vi "Example1 Chap1.vi"() -> ()   [LabVIEW 2013]
panel:
  in  "stop":bool
  out "Gauge":i32(knob) scale=0.0..10.0
  in  "Start":bool
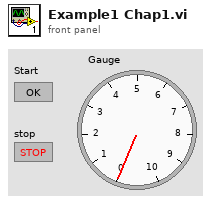
[diagram p1: front panel]
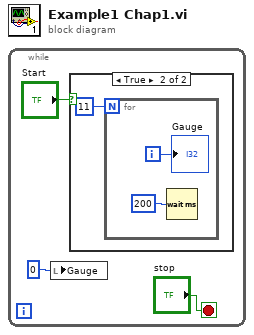
[diagram p0: block diagram]
diagram:
  n1 = while {
    stop <- "stop" stop-if-true
    n2 = local write "Gauge"(0) -> ()
    n3 = case shown="True" "Start" {
      frame False {
      }
      frame True {
        n4 = for {
          N: 11 ("Numeric") -> [_]
          i -> [w5]
          n5 = Wait (ms)(milliseconds to wait=u32 200) -> ()  [unwired: 1 out]
          "Gauge" <- w5
        }
      }
    }
  }
